vi "Add Response_Byte count.vi"(6 "Channel refnum":T1=18446744073709551615 format="%.0x", 7 "Byte Count value":u32, 8 "error in (no error)":errorcluster, 11 "Response refnum in":T1=18446744073709551615 format="%.0x") -> (0 "error out":errorcluster, 3 "Response refnum out":T1=18446744073709551615 format="%.0x")   [LabVIEW 2019, in "Scripting API.lvlib"]
uses:
  Scripting API.lvlib
  <vilib>/NI VeriStand/Custom Device API/Custom Device Item Ref.ctl
  <vilib>/NI VeriStand/Custom Device API/Custom Device API.lvlib
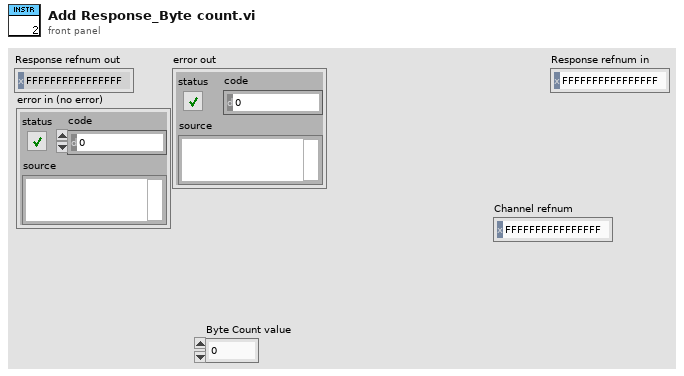
[diagram p1: front panel]
types:
  T1 = typedef "Custom Device API.lvlib/Custom Device Item Ref.ctl" = u64
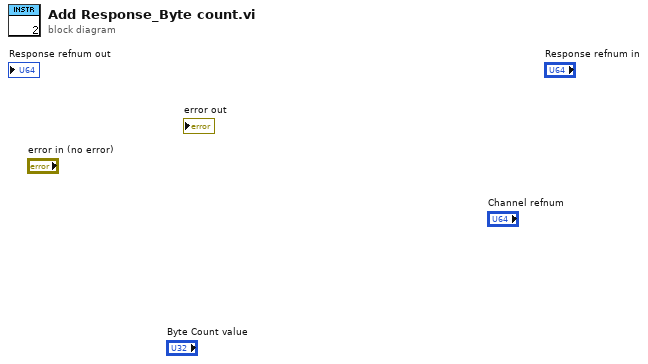
[diagram p0: block diagram]
diagram:
